vi "U3 Single AIN.vi"(8 "error in":errorcluster, 10 "Channel #":i32) -> (0 "error out":errorcluster, 2 "Binary Value Read":dbl format="%.6f")   [LabVIEW 2021]
panel:
  out "Data Read":u8[](array[numeric]) format="%.0x"
  # "Aquires 1 analog input channel from the first found U3."
  # "Use 0-7"
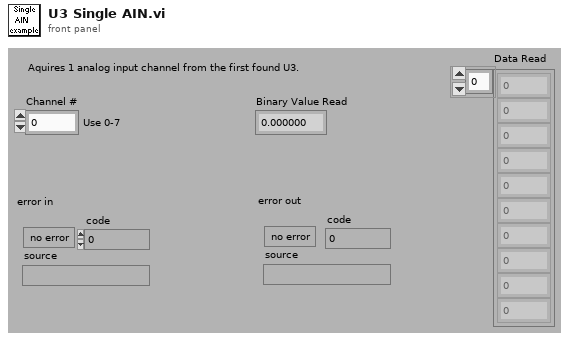
[diagram p1: front panel]
types:
  T1 = cluster{"Open LabJack":bool, "Address":string, "FirstFound":bool}
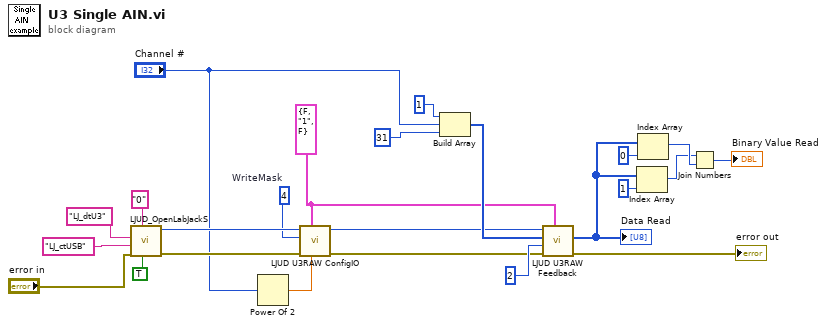
[diagram p0: block diagram]
diagram:
  w3 = u8 4  # WriteMask
  w16 = T1 {"Open LabJack"=FALSE, "Address"="1", "FirstFound"=FALSE} ("Comm Settings")
  n1 = call "LJUD_OpenLabJackS.vi"("FirstFound"=TRUE, "Address"="0", "error in"="error in", "ConnectionType"="LJ_ctUSB", "DeviceType"="LJ_dtU3") -> ("error out"=w15:errorcluster, "Handle"=w17:i32)  [unwired: 4 in, 1 out]
  n2 = Power Of 2(x="Channel #") -> (2^x=w1:dbl)
  n3 = call "LJUD U3RAW ConfigIO.vi"("FIOAnalog"=w1, "Comm Settings"=w16, "error in (no error)"=w15, "WriteMask"=w3, "Handle In"=w17) -> ("error out"=w14:errorcluster, "Handle Out"=w13:i32)  [unwired: 5 in]
  n4 = Build Array(u8 1 ("Input Element"), "Channel #", 31 ("Input Element")) -> (w19:i32[])
  n5 = call "LJUD U3RAW Feedback.vi"("Comm Settings"=w16, "error in (no error)"=w14, "# Data Bytes to Read"=2, "Data"=w19, "Handle In"=w13) -> ("error out"=→"error out":errorcluster, "Data Read"=w7:u8[])  [unwired: 4 in, 1 out]
  "Data Read" <- w7
  n6 = Index Array(array=w7, index=1 ("Index")) -> (element=w5:u8)
  n7 = Index Array(array=w7, index=0 ("Index")) -> (element=w11:u8)
  n8 = Join Numbers(hi=w5, lo=w11) -> ((hi.lo)=→"Binary Value Read":u16)
